vi "Synchronize to RT (RT Host) - cRIO.vi"() -> ()   [LabVIEW 2010]
uses:
  <vilib>/rvi/interface/nirviOpenFPGA/nirviOpenFPGA.xnode
  FPGA Timekeeper.lvlib
  <vilib>/userDefined/High Color/nirio_resource_hc.ctl
  <vilib>/rvi/interface/nirviReadWriteControl/nirviReadWriteControl.xnode
  <vilib>/rvi/interface/nirviCloseFPGA/nirviCloseFPGA.xnode
  <vilib>/FPGAPlugInAG/Dynamic/niLvFpga_Close_Dynamic.vi
  NiFpgaLv.dll
  <vilib>/Utility/error.llb/Error Cluster From Error Code.vi
  <vilib>/rvi/errors/niLvFpgaWhatHappensToTopLevelVI.ctl
  <vilib>/rvi/interface/common/niFpgaNodeNameForErrorReporting.ctl
  <vilib>/rvi/errors/niLvFpgaAdjustHostInterfaceError.vi
  Synchronize to RT (FPGA) - cRIO.vi
panel:
  out "error out":errorcluster
  in  "stop":bool
  out "offset from RT time (ns)":i32
  out "FPGA Timekeeper locked":bool
  # "This example synchronizes the FPGA Timekeeper on a CompactRIO FPGA target with the current system time of a Real-Time target."
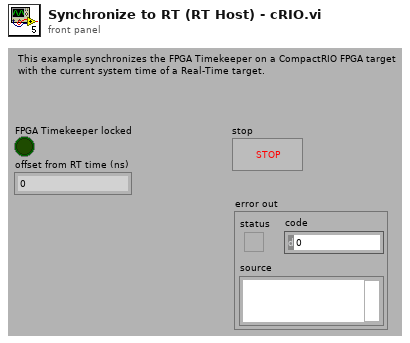
[diagram p1: front panel]
types:
  T1 = typedef "niFpgaNodeNameForErrorReporting.ctl" = enum16{"Open FPGA VI Reference", "Read/Write Control", "Invoke Method: Abort", "Invoke Method: Acknowledge IRQ", "Invoke Method: Download", "Invoke Method: FIFO.Configure", "Invoke Method: FIFO.Read", "Invoke Method: FIFO.Start", "Invoke Method: FIFO.Stop", "Invoke Method: FIFO.Write", "Invoke Method: Reset", "Invoke Method: Run", "Invoke Method: Wait on IRQ", "Close FPGA VI Reference"}
  T2 = typedef "niLvFpgaWhatHappensToTopLevelVI.ctl" = enum16{"top level VI scripted behind XNode", "top level VI inlined behind XNode"}
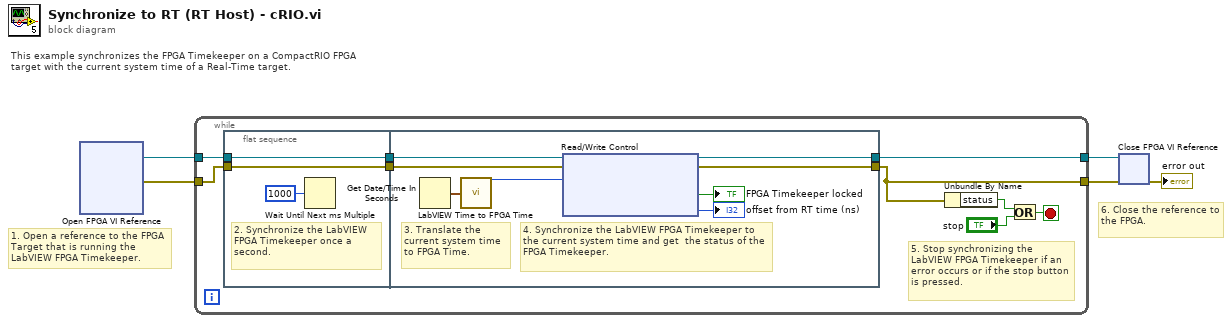
[diagram p0: block diagram]
diagram:
  # "This example synchronizes the FPGA Timekeeper on a CompactRIO FPGA target with the current system time of a Real-Time target."
  # "6. Close the reference to the FPGA."
  # "1. Open a reference to the FPGA\nTarget that is running the \nLabVIEW FPGA Timekeeper."
  n1 = xnode "Open FPGA VI Reference"() -> ("FPGA VI Reference Out"=w5:refnum<k20>, "error out"=w4:errorcluster)  [unwired: 2 in]
  n2 = while {
    tunnel: w5 -> [w14]
    tunnel: w4 -> [w9]
    tunnel: [w13] -> w3
    tunnel: [w7] -> w1
    stop <- w11 stop-if-true
    # "5. Stop synchronizing the LabVIEW FPGA Timekeeper if an error occurs or if the stop button is pressed."
    n3 = flat-sequence {
      tunnel: w14 -> [w17]
      tunnel: [w17] -> w10
      tunnel: w9 -> [w16]
      tunnel: [w16] -> w8
      tunnel: [w25] -> w13
      tunnel: w10 -> [w22]
      tunnel: w8 -> [w21]
      tunnel: [w18] -> w7
      frame #0 {
        # "2. Synchronize the LabVIEW FPGA Timekeeper once a second."
        n4 = Wait Until Next ms Multiple(millisecond multiple=u32 1000) -> ()  [unwired: 1 out]
      }
      frame #1 {
        # "4. Synchronize the LabVIEW FPGA Timekeeper to the current system time and get  the status of the FPGA Timekeeper."
        # "3. Translate the current system time to FPGA Time."
        n5 = Get Date/Time In Seconds() -> (seconds since 1Jan1904=w20:timestamp)
        n6 = call "LabVIEW Time to FPGA Time.vi"("LabVIEW time"=w20) -> ("FPGA time (ns)"=w19:u64)
        n7 = xnode "Read/Write Control"("FPGA VI Reference In"=w22, "error in"=w21, "RT time (ns)"=w19) -> ("FPGA VI Reference Out"=w25:refnum<k20>, "error out"=w18:errorcluster, "FPGA Timekeeper locked"=→"FPGA Timekeeper locked":bool, "offset from RT time (ns)"=→"offset from RT time (ns)":i32)
      }
    }
    n8 = Unbundle By Name(w7) -> ("status"=w6:bool)
    n9 = Or(x=w6, y="stop") -> (x .or. y?=w11:bool)
  }
  n10 = xnode "Close FPGA VI Reference"("FPGA VI Reference In"=w3, "error in"=w1) -> ("error out"=→"error out":errorcluster)
